vi "SubVI_Factorial.vi"(0 "Input":i32) -> (4 "Factorial":i32)   [LabVIEW 2025]
panel:
  # "Finding Factorial of Input"
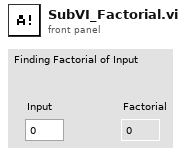
[diagram p1: front panel]
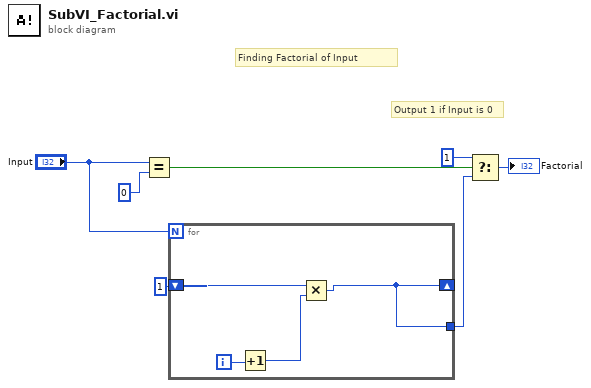
[diagram p0: block diagram]
diagram:
  # "Output 1 if Input is 0"
  # "Finding Factorial of Input"
  n1 = Equal?(x="Input", y=0) -> (x = y?=w5:bool)
  n2 = for {
    N: "Input" -> [_]
    shift-right: [w8] -> _
    shift-left: 1 -> [w9]
    tunnel: [w8] -> w4
    i -> [w11]
    n3 = Increment(x=w11) -> (x+1=w10:i32)
    n4 = Multiply(x=w9, y=w10) -> (x*y=w8:i32)
  }
  n5 = Select(t=1, s=w5, f=w4) -> (s? t:f=→"Factorial":i32)
